vi "Read Error log file.vi"(8 "error in (no error)":errorcluster, 11 "Error Log in":refnum<class "Error Log.lvclass">) -> (0 "error out":errorcluster, 2 "Error log file":path, 3 "Error Log out":refnum<class "Error Log.lvclass">)   [LabVIEW 2020, in "Error Log.lvclass"]
uses:
  Error Log.lvclass
  Error Log.lvclass/Error Log.ctl
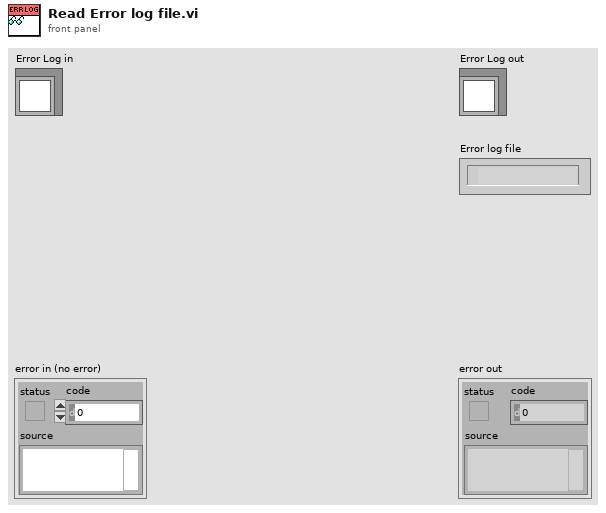
[diagram p1: front panel]
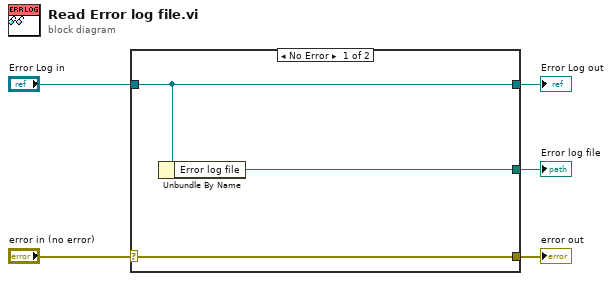
[diagram p0: block diagram]
diagram:
  n1 = case shown="No Error" "error in (no error)" {
    selector: "error in (no error)" -> [w8 w9]
    tunnel: [w8 w9] -> w4
    tunnel: [w7 w10] -> w2
    tunnel: "Error Log in" -> [w7 w10]
    tunnel: [w6 _] -> w1
    frame No Error {
      n2 = Unbundle By Name(w7) -> ("Error log file"=w6:path)
    }
    frame Error {
    }
  }
  "error out" <- w4
  "Error Log out" <- w2
  "Error log file" <- w1
